vi "Temperature Warnings.vi"() -> ()   [LabVIEW 2015]
doc: "This VI is used to determine the string to output to the weather station based on the current temperature and limit settings.\n\nInputs: Current Temperature (DBL), Minimum Temperature (DBL), and Maximum Temperature (DBL).\nOutputs: Warning Text (string) and Warning? (Boolean)."
panel:
  out "Error Out":errorcluster
  in  "Error In":errorcluster
  out "Warning Text":string="No Warning"
  out "Warning?":bool
  in  "Min Temperature":dbl
  in  "Max Temperature":dbl
  in  "Current Temperature":dbl
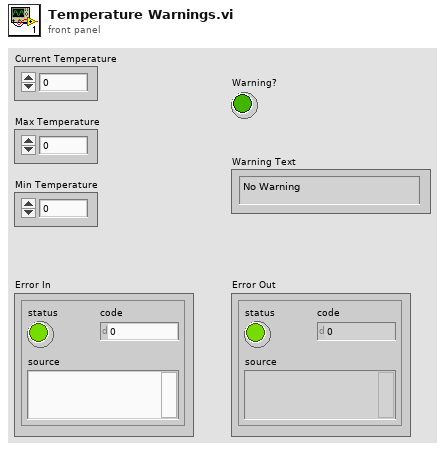
[diagram p1: front panel]
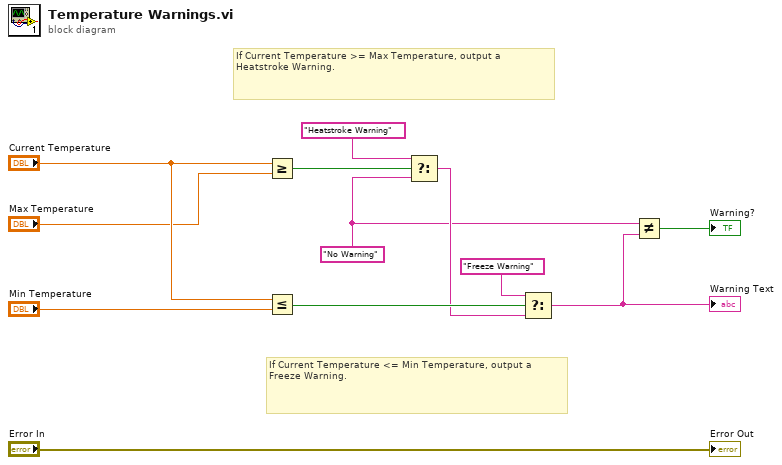
[diagram p0: block diagram]
diagram:
  w2 = "No Warning" ("f")
  # "If Current Temperature >= Max Temperature, output a Heatstroke Warning."
  # "If Current Temperature <= Min Temperature, output a Freeze Warning."
  n1 = Greater Or Equal?(x="Current Temperature", y="Max Temperature") -> (x >= y?=w7:bool)
  n2 = Less Or Equal?(x="Current Temperature", y="Min Temperature") -> (x <= y?=w4:bool)
  n3 = Select(t="Heatstroke Warning", s=w7, f=w2) -> (s? t:f=w3:string)
  n4 = Select(t="Freeze Warning", s=w4, f=w3) -> (s? t:f=w8:string)
  "Warning Text" <- w8
  n5 = Not Equal?(x=w2, y=w8) -> (x != y?=→"Warning?":bool)
  "Error Out" <- "Error In"
